vi "Read Error Message.vi"(8 "error in (no error)":errorcluster, 11 "httpRequest in":refnum<class "httpResponse.lvclass">) -> (0 "error out":errorcluster, 2 "error-message":string, 3 "httpRequest out":refnum<class "httpResponse.lvclass">)   [LabVIEW 2020]
uses:
  httpResponse.lvclass/httpResponse.ctl
  httpResponse.lvclass
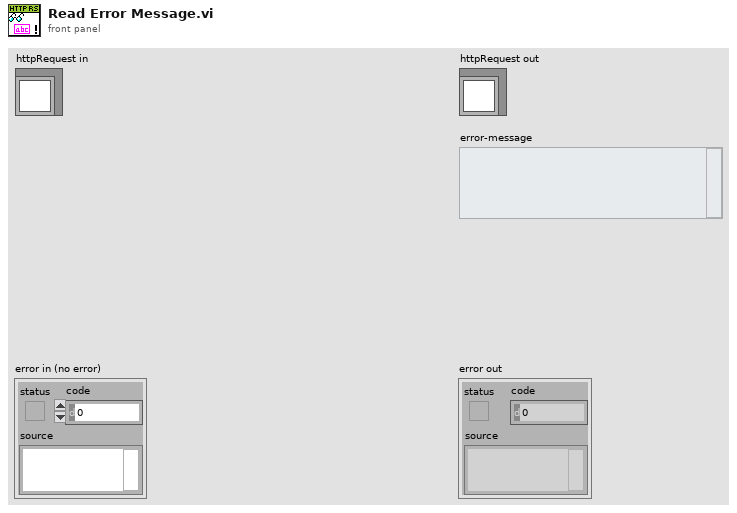
[diagram p1: front panel]
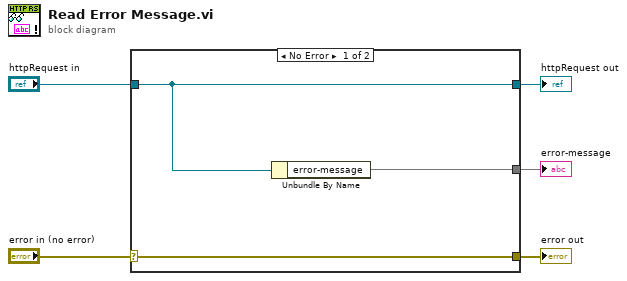
[diagram p0: block diagram]
diagram:
  n1 = case shown="No Error" "error in (no error)" {
    selector: "error in (no error)" -> [w8 w9]
    tunnel: [w8 w9] -> w4
    tunnel: [w7 w10] -> w2
    tunnel: "httpRequest in" -> [w7 w10]
    tunnel: [w6 _] -> w1
    frame No Error {
      n2 = Unbundle By Name(w7) -> ("error-message"=w6)
    }
    frame Error {
    }
  }
  "error out" <- w4
  "httpRequest out" <- w2
  "error-message" <- w1
